vi "TT Settings Dialog.vi"(8 "error in (no error)":errorcluster, 11 "TT Module Config in":T2) -> (0 "error out":errorcluster, 1 "Cancelled?":bool=TRUE, 2 "UI Refresh Needed?":bool, 3 "TT Module Config out":T2)   [LabVIEW 2018, in "TT Module.lvlib"]
doc: "Dialog for selecting user specified settings."
uses:
  TT Module.lvlib
  Controls/TT Module Config Cluster.ctl
  <vilib>/Utility/miscctls.llb/LVPoint32TypeDef.ctl
  Tag VIs/Numeric Alarm Settings Cluster.ctl
  PT Module/Controls/PT Settings Dialog.ctl
  Tag VIs/Tag FGV Operation Enum.ctl
  Shared Variables/Simple Alarm Values Cluster.ctl
  Shared Variables/Dynamic Shared Variables.lvlib
  PT Module/PT Module.lvlib
panel:
  in  "Module Name":string
  in  "Settings Dialog":T1 {"Input Channel Tag Name" items=["Temperature", "Temperature_0"]}
  in  "Cancel Button":bool
  in  "OK Button":bool
  # "Non visible portion of dialog (needed for connector pane)."
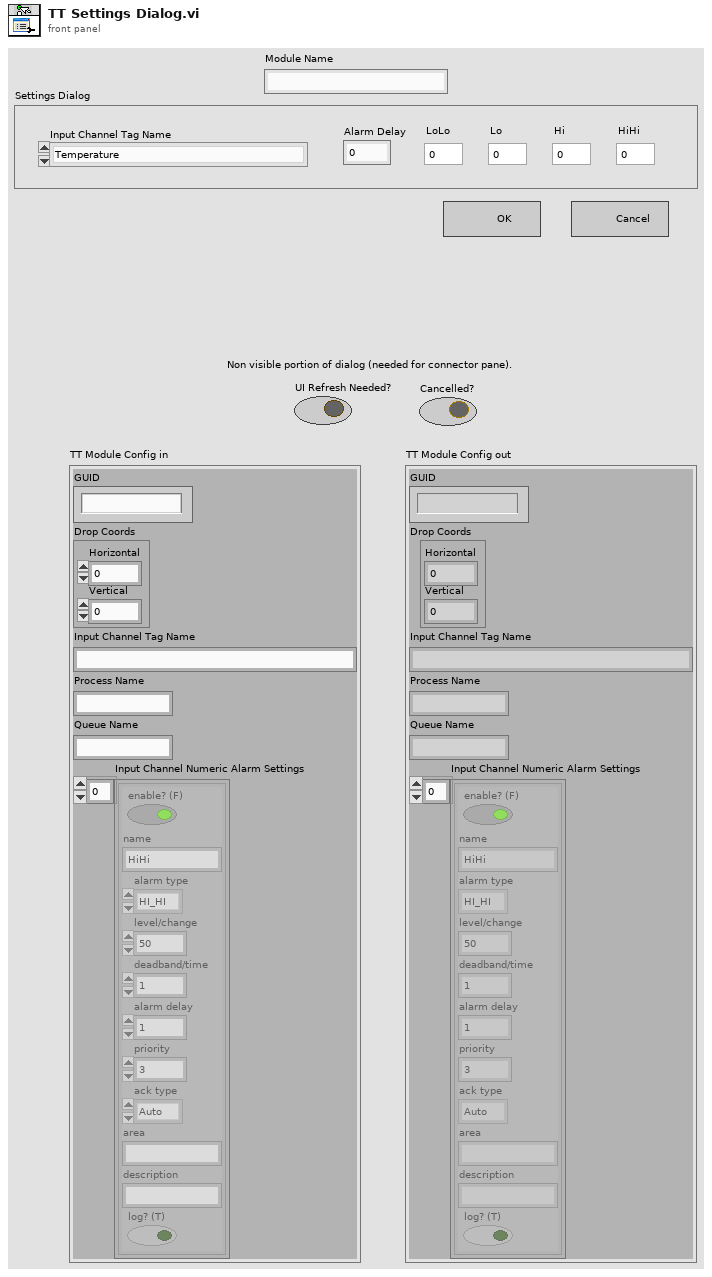
[diagram p1: front panel]
types:
  T1 = typedef "PT Module.lvlib/PT Settings Dialog.ctl" = cluster{"Input Channel Tag Name":u16, "LoLo":dbl, "Lo":dbl, "Hi":dbl, "HiHi":dbl, "Alarm Delay":dbl}
  T2 = typedef "TT Module.lvlib/TT Module Config Cluster.ctl" = cluster{"GUID":string, "Drop Coords":T3, "Input Channel Tag Name ":string, "Process Name":string, "Queue Name":string, "Input Channel Numeric Alarm Settings":T4[]}
  T3 = typedef "LVPoint32TypeDef.ctl" = cluster{"Horizontal":i32, "Vertical":i32}
  T4 = typedef "Numeric Alarm Settings Cluster.ctl" = cluster{"enable? (F)":bool, "name":string, "alarm type":enum16{"HI_HI", "HI", "LO", "LO_LO"}, "level/change":dbl, "deadband/time":dbl, "alarm delay":dbl, "priority":u32, "ack type":enum16{"Auto", "User", "None", "Each Occurrence"}, "area":string, "description":string, "log? (T)":bool}
  T5 = typedef "Tag FGV Operation Enum.ctl" = enum16{"Init", "Set Notification Queue", "Create Tag", "Commit", "Write Tag (Numeric)", "Write Tag (Boolean)", "Read All Tags", "Read One Tag", "Delete Tag Category", "Set Alarm Parameters (Numeric)", "Set Alarm Parameters (Boolean)", "Enable All Alarms", "Disable All Alarms", "Delete All Tags", "Read Alarms", "Ack Alarm", "Read Alarm Parameters (Numeric)", "Read Alarm Parameters (Boolean)"}
  T6 = typedef "Dynamic Shared Variables.lvlib/Simple Alarm Values Cluster.ctl" = cluster{"tag name":string, "HiHi":dbl, "Hi":dbl, "Lo":dbl, "LoLo":dbl, "alarm delay":dbl}
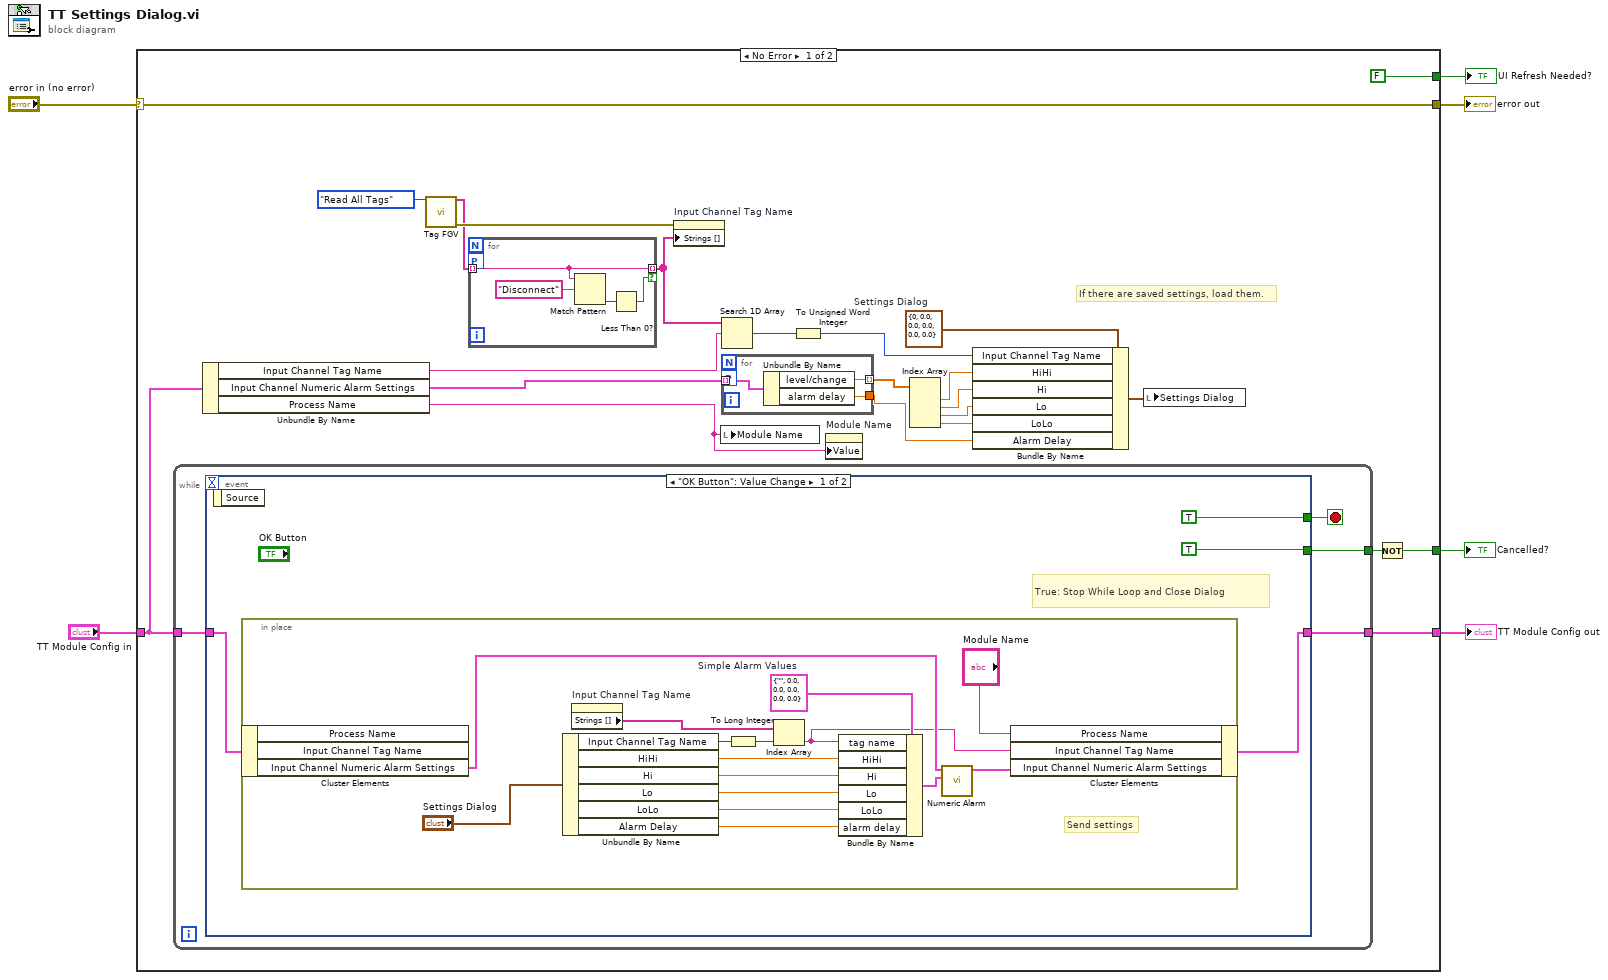
[diagram p0: block diagram]
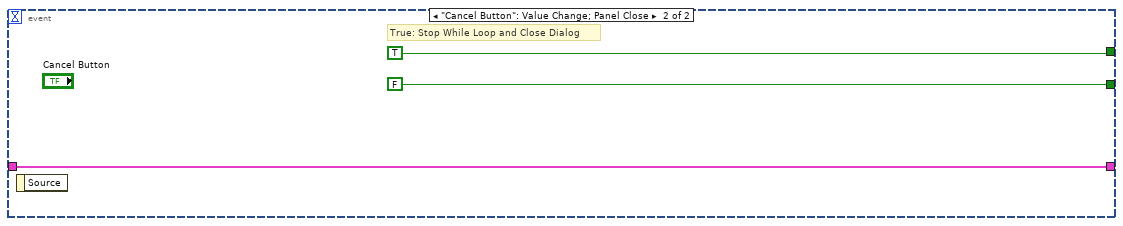
[diagram p2: hidden frame]
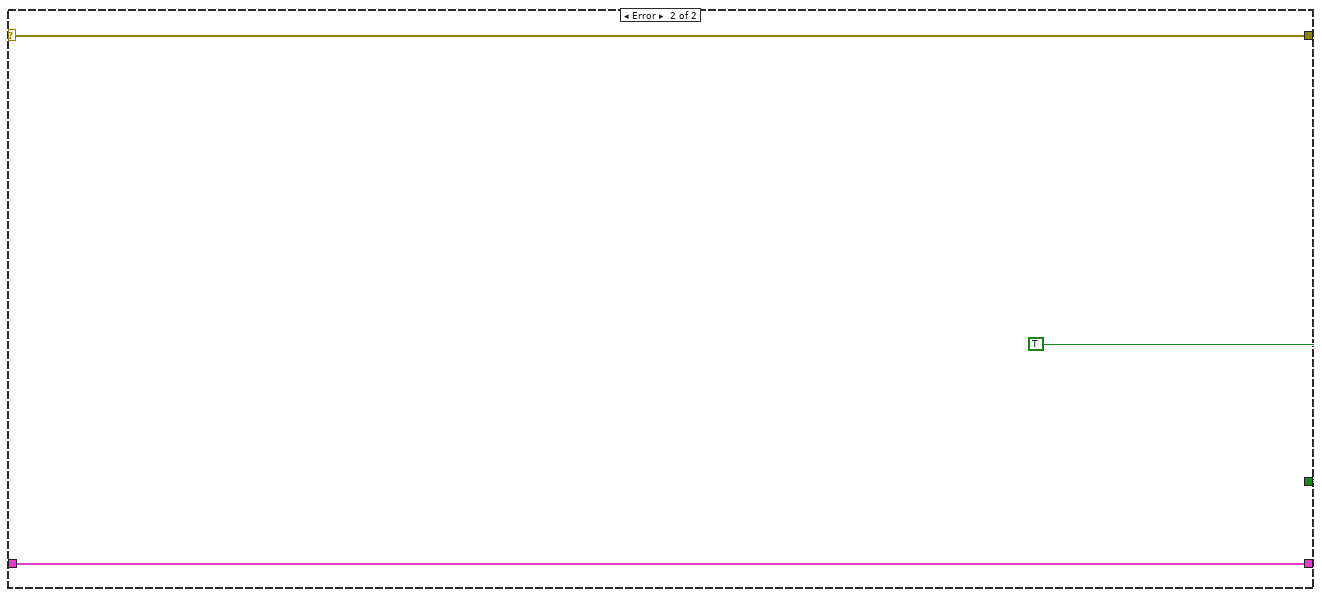
[diagram p3: hidden frame]
diagram:
  n1 = case shown="No Error" "error in (no error)" {
    selector: "error in (no error)" -> [w29 w65]
    tunnel: [w29 w65] -> w6
    tunnel: "TT Module Config in" -> [w26 w64]
    tunnel: [w27 w64] -> w1
    tunnel: [FALSE ("UI Refresh Needed?") _] -> w4
    tunnel: [w24 TRUE ("UI Refresh Needed?")] -> w3
    frame No Error {
      w20 = T1 {"Input Channel Tag Name"=0, "LoLo"=0.0, "Lo"=0.0, "Hi"=0.0, "HiHi"=0.0, "Alarm Delay"=0.0}  # Settings Dialog
      # "If there are saved settings, load them."
      n2 = while {
        tunnel: [w40] -> w25
        tunnel: [w37] -> w27
        tunnel: w26 -> [w39]
        stop <- w38 stop-if-true
        n3 = event shown="[0] \"OK Button\": Value Change" {
          selector: _ -> [_ _]
          dyn-events: _ -> [_ _]
          timeout: _ -> [_ _]
          tunnel: w39 -> [w42 w62]
          tunnel: [TRUE ("UI Refresh Needed?") FALSE ("UI Refresh Needed?")] -> w40
          tunnel: [TRUE TRUE] -> w38
          tunnel: [w41 w62] -> w37
          event "OK Button": Value Change {
            # "True: Stop While Loop and Close Dialog"
            n4 = event-data() -> ()  [unwired: 1 in, 1 out]
            n5 = in-place {
              w51 = T6 {"tag name"="", "HiHi"=0.0, "Hi"=0.0, "Lo"=0.0, "LoLo"=0.0, "alarm delay"=0.0}  # Simple Alarm Values
              # "Send settings"
              n6 = in-place-cluster #1(w42) -> ("Input Channel Numeric Alarm Settings"=w48:T4[])  [unwired: 2 out]
              n7 = Unbundle By Name("Settings Dialog") -> ("Input Channel Tag Name"=w57:u16, "HiHi"=w55:dbl, "Hi"=w54:dbl, "Lo"=w53:dbl, "LoLo"=w52:dbl, "Alarm Delay"=w49:dbl)
              n8 = property on="Input Channel Tag Name" class="Ring (strict)"() -> ("Strings []"=w58:string[])  [unwired: 2 in, 2 out]
              n9 = To Long Integer(number=w57) -> (32bit integer=w56:i32)
              n10 = Index Array(array=w58, index=w56) -> (element=w46:string)
              n11 = Bundle By Name(cluster=w51, "tag name"=w46, "HiHi"=w55, "Hi"=w54, "Lo"=w53, "LoLo"=w52, "alarm delay"=w49) -> (w50:T6)
              n12 = call "Numeric Alarm.vi"("Simple Alarm Values"=w50, "Alarms in"=w48) -> ("Alarms out"=w45:T4[])  [unwired: 9 in]
              n13 = in-place-cluster #1("Process Name"="Module Name", "Input Channel Tag Name"=w46, "Input Channel Numeric Alarm Settings"=w45) -> (w41:T2)
            }
          }
          event "Cancel Button": Value Change; Panel Close {
            # "True: Stop While Loop and Close Dialog"
            n14 = event-data() -> ()  [unwired: 1 in, 1 out]
          }
        }
      }
      n15 = Unbundle By Name(w26) -> ("Input Channel Tag Name"=w23:string, "Input Channel Numeric Alarm Settings"=w21:T4[], "Process Name"=w12:string)
      n16 = call "Tag FGV.vi"("Operation"=Tag_FGV_Operation_Enum."Read All Tags") -> ("Tag Names"=w9:string[], "error out"=w10:errorcluster)  [unwired: 7 in, 6 out]
      n17 = for {
        tunnel: w9 -> [w31] mode=indexing
        tunnel: [w31] -> w8 mode=indexing if=w30
        workers-P: _ -> [_]
        n18 = Match Pattern(string=w31, regular expression="Disconnect" ("name")) -> (offset past match=w33:i32)  [unwired: 1 in, 3 out]
        n19 = Less Than 0?(x=w33) -> (x < 0?=w30:bool)
      }
      n20 = property on="Input Channel Tag Name" class="Ring (strict)"(error in=w10, "Strings []"=w8) -> ()  [unwired: 1 in, 2 out]
      n21 = local write "Module Name"(w12) -> ()
      n22 = Search 1D Array(1D array=w8, element=w23) -> (index of element=w22:i32)  [unwired: 1 in]
      n23 = for {
        tunnel: w21 -> [w36] mode=indexing
        tunnel: [w35] -> w17 mode=indexing
        tunnel: [w34] -> w7
        workers-P: _ -> [_]
        n24 = Unbundle By Name(w36) -> ("level/change"=w35:dbl, "alarm delay"=w34:dbl)
      }
      n25 = To Unsigned Word Integer(number=w22) -> (unsigned 16bit integer=w19:u16)
      n26 = property on="Module Name" class="Str"("Value"=w12) -> ()  [unwired: 2 in, 2 out]
      n27 = Index Array(array=w17) -> (element #1=w16:dbl, element #2=w15:dbl, element #3=w14:dbl, element #4=w13:dbl)  [unwired: 4 in]
      n28 = Bundle By Name(cluster=w20, "Input Channel Tag Name"=w19, "HiHi"=w16, "Hi"=w15, "Lo"=w14, "LoLo"=w13, "Alarm Delay"=w7) -> (w18:T1)
      n29 = local write "Settings Dialog"(w18) -> ()
      n30 = Not(x=w25) -> (.not. x?=w24:bool)
    }
    frame Error {
    }
  }
  "UI Refresh Needed?" <- w4
  "error out" <- w6
  "TT Module Config out" <- w1
  "Cancelled?" <- w3
